vi "Run Short Check.vi"(8 "error in":errorcluster, 10 "Position":u32, 11 "Driver Test in":refnum<class "Driver Test.lvclass">) -> (0 "error out":errorcluster, 3 "Protected":bool)   [LabVIEW 2015, in "Short Check.lvclass"]
uses:
  Short Check.lvclass
  Driver Test/Driver Test.lvclass
  CBTF Applications/Driver Board Testing/Main/Application/Application/Class/typedefs/Instrument Selector -- Enum.ctl
  Classes/Instruments/AC Power Supply/AC Power Supply/Class/AC Power Supply.lvclass
  CBTF Applications/Driver Board Testing/Main/Application/Application/Class/Driver Board Test.lvclass
  Test Class/Test Class.lvclass
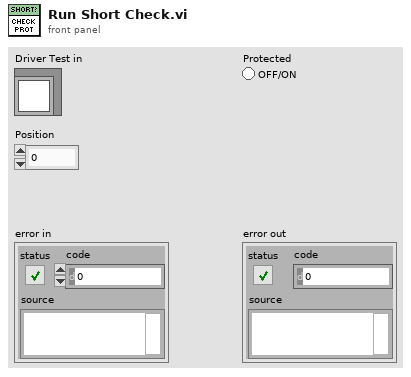
[diagram p1: front panel]
types:
  T1 = typedef "Driver Board Test.lvlib/Driver Board Test.lvclass/Instrument Selector -- Enum.ctl" = enum16{"ACPS1", "ACPS2", "DCPS1", "DCPS2", "DCPS3", "DCLoad1", "DCLoad2", "DPM1", "DPM2", "Switch1", "PXI1Slot2", "PXI1Slot3", "cDAQ1Mod5", "cDAQ1Mod6", "cDAQ1Mod7", "cDAQ1Mod8", "cDAQ1Mod1", "cDAQ1Mod2", "cDAQ1Mod3", "cDAQ1Mod4", "cDAQ2Mod1", "cDAQ2Mod2", "cDAQ2Mod3", "cDAQ2Mod4"}
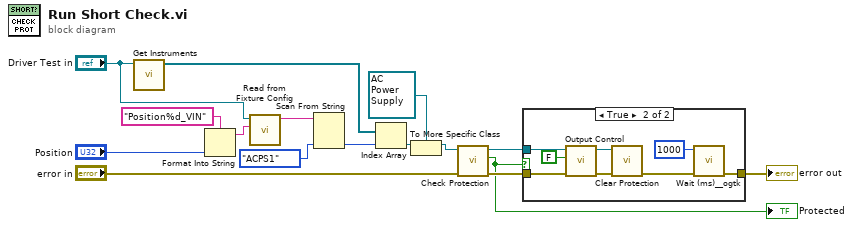
[diagram p0: block diagram]
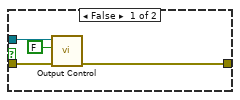
[diagram p2: hidden frame]
diagram:
  n1 = call "Get Instruments.vi"("Test Class in"="Driver Test in") -> ("Instruments"=w4:refnum<class "Instrument.lvclass">[])  [unwired: 9 in, 1 out]
  n2 = Format Into String(format string="Position%d_VIN", "Position") -> (resulting string=w11:string)  [unwired: 2 in, 1 out]
  n3 = call-dynamic "Read from Fixture Config.vi"("Key"=w11, "Test Class in"="Driver Test in") -> ("Instrument Info"=w10:string)  [unwired: 8 in, 1 out]
  n4 = Scan From String(input string=w10, default 1=Instrument_Selector_--_Enum."ACPS1" ("Instrument")) -> (output 1=w7:T1)  [unwired: 3 in, 3 out]
  n5 = Index Array(array=w4, index=w7) -> (element=w6:refnum<class "Instrument.lvclass">)
  n6 = To More Specific Class(target class=refnum<class "AC Power Supply.lvclass"> refnum ("AC Power Supply in"), reference=w6) -> (specific class reference=w2:refnum<class "AC Power Supply.lvclass">)  [unwired: 1 in, 1 out]
  n7 = call-dynamic "Check Protection.vi"("error in (no error)"="error in", "AC Power Supply in"=w2) -> ("error out"=w14:errorcluster, "Protection"=w13:bool, "AC Power Supply out"=w15:refnum<class "AC Power Supply.lvclass">)  [unwired: 7 in]
  "Protected" <- w13
  n8 = case shown="True" w13 {
    tunnel: w15 -> [w18 w28]
    tunnel: w14 -> [w19 w25]
    tunnel: [w17 w21] -> w12
    frame False {
      n9 = call-dynamic "Output Control.vi"("error in (no error)"=w19, "Enabled"=FALSE, "Acrobat Template in"=w18) -> ("error out"=w17:errorcluster)  [unwired: 7 in, 1 out]
    }
    frame True {
      n10 = call-dynamic "Output Control.vi"("error in (no error)"=w25, "Enabled"=FALSE, "Acrobat Template in"=w28) -> ("error out"=w24:errorcluster, "Acrobat Template out"=w26:refnum<class "AC Power Supply.lvclass">)  [unwired: 7 in]
      n11 = call-dynamic "Clear Protection.vi"("error in (no error)"=w24, "Acrobat Template in"=w26) -> ("error out"=w23:errorcluster)  [unwired: 8 in, 1 out]
      n12 = call <userlib>:"Wait (ms)__ogtk.vi"("error in (no error)"=w23, "milliseconds to wait"=u32 1000) -> ("error out"=w21:errorcluster)  [unwired: 8 in, 1 out]
    }
  }
  "error out" <- w12
